vi "Create.vi"(10 "Position":T1) -> (3 "Snake out":refnum<class "Snake.lvclass">)   [LabVIEW 2020, in "Snake.lvclass"]
uses:
  Snake.lvclass
  Particle/Position.ctl
  Snake.lvclass/Snake.ctl
  Particle.lvclass
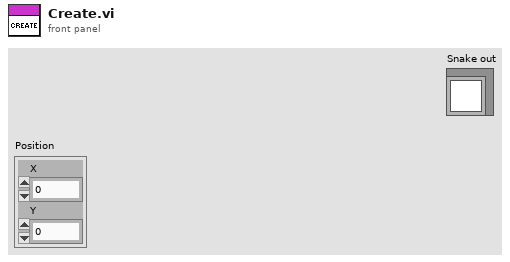
[diagram p1: front panel]
types:
  T1 = typedef "Particle.lvclass/Position.ctl" = cluster{"X":i32, "Y":i32}
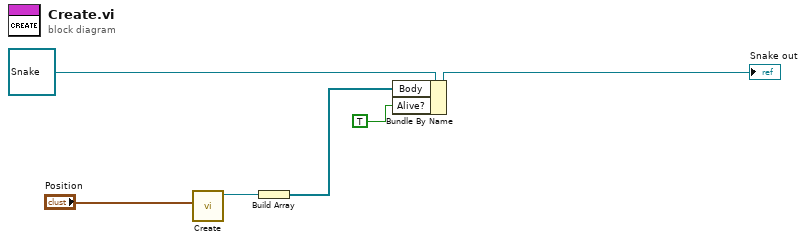
[diagram p0: block diagram]
diagram:
  n1 = call "Create.vi"("Position"="Position") -> ("Particle out"=w3:refnum<class "Particle.lvclass">)  [unwired: 10 in]
  n2 = Build Array(w3) -> (w2:refnum<class "Particle.lvclass">[])
  n3 = Bundle By Name(cluster=refnum<class "Snake.lvclass"> refnum ("Snake in"), "Body"=w2, "Alive?"=TRUE) -> (→"Snake out":refnum<class "Snake.lvclass">)
